vi "timer.vi"(8 "Time Duration":dbl, 11 "Enum":T1) -> (2 "Time Elapsed":dbl, 5 "Time Elapsed?":bool)   [LabVIEW 2020]
uses:
  timer states.ctl
panel:
  # "Keep in mind that an action engine uses shift register to store values, \nso its execution mode needs to be set to non-reentrant."
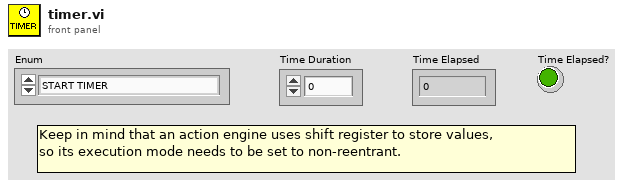
[diagram p1: front panel]
types:
  T1 = typedef "timer states.ctl" = enum16{"START TIMER", "RESTART TIMER", "CHECK TIMER", "PAUSE TIMER"}
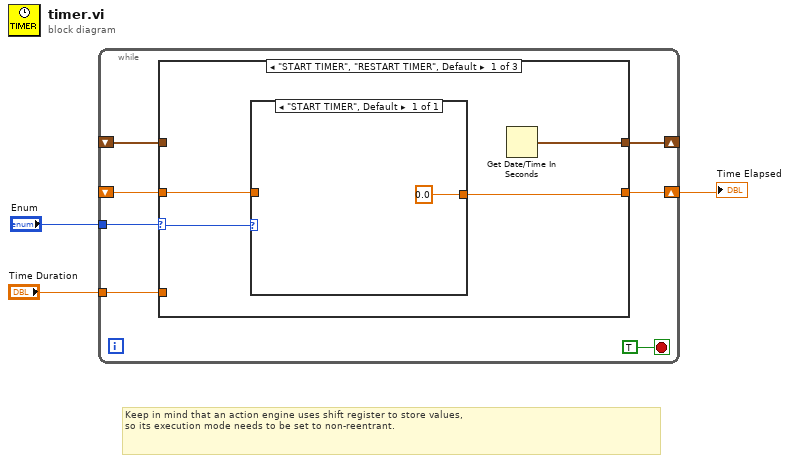
[diagram p0: block diagram]
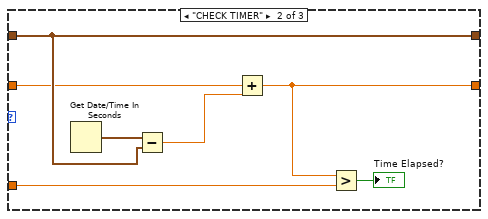
[diagram p2: hidden frame]
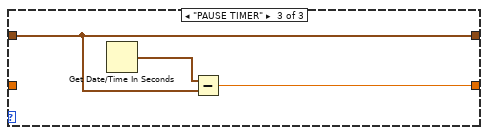
[diagram p3: hidden frame]
diagram:
  # "Keep in mind that an action engine uses shift register to store values, \nso its execution mode needs to be set to non-reentrant."
  n1 = while {
    tunnel: "Enum" -> [w10]
    shift-right: [w4] -> _
    shift-left: _ -> [w5]
    shift-right: [w8] -> w1
    shift-left: _ -> [w7]
    tunnel: "Time Duration" -> [w9]
    stop <- TRUE stop-if-true
    n2 = case shown="\"START TIMER\", \"RESTART TIMER\", Default" w10 {
      selector: w10 -> [w14 _ _]
      tunnel: w9 -> [_ w18 _]
      tunnel: [w13 w17 w23] -> w8
      tunnel: w7 -> [w12 w20 _]
      tunnel: w5 -> [_ w21 w24]
      tunnel: [w11 w21 w24] -> w4
      frame "START TIMER", "RESTART TIMER", Default {
        n3 = case shown="\"START TIMER\", Default" w14 {
          tunnel: [0.0] -> w13
          tunnel: w12 -> [_]
          frame "START TIMER", Default {
          }
        }
        n4 = Get Date/Time In Seconds() -> (seconds since 1Jan1904=w11:timestamp)
      }
      frame "CHECK TIMER" {
        n5 = Get Date/Time In Seconds() -> (seconds since 1Jan1904=w22:timestamp)
        n6 = Subtract(x=w22, y=w21) -> (x-y=w19:dbl)
        n7 = Add(x=w20, y=w19) -> (x+y=w17:dbl)
        n8 = Greater?(x=w17, y=w18) -> (0:→"Time Elapsed?":bool)
      }
      frame "PAUSE TIMER" {
        n9 = Get Date/Time In Seconds() -> (seconds since 1Jan1904=w25:timestamp)
        n10 = Subtract(x=w25, y=w24) -> (x-y=w23:dbl)
      }
    }
  }
  "Time Elapsed" <- w1
